vi "Do Core.vi"(8 "error in (no error)":errorcluster, 10 "Actor in":refnum<class "Actor.lvclass">, 11 "Ack Completion Long Exec Meth Msg in":refnum<class "Ack Completion with Error Msg.lvclass">) -> (0 "error out":errorcluster, 2 "Actor out":refnum<class "Actor.lvclass">)   [LabVIEW 2023, in "Async Methods Actor Example.lvlib" / "Ack Completion with Error Msg.lvclass"]
doc: "(<B>Filename</B>: Actor Framework.lvlib:Message.lvclass:Do.vi)\n\nDefines what a message does when it is received by an actor. Generally, a message instructs an actor to invoke one of its methods. By default, this method does nothing. A child class must override it to define behavior. Create a child class by using the Actor Framework Message Maker dialog box."
uses:
  Ack Completion with Error Msg.lvclass
  C:/Program Files/National Instruments/LabVIEW 2023/vi.lib/LS Instruments AG/Async Methods Actor/Async Methods Actor/Async Methods Actor Messages/Completion Notification Msg/Completion Notification Msg.lvclass
  <vilib>/ActorFramework/Actor/Actor.lvclass
  Async Methods Actor Example/Async Methods Actor Example.lvclass
  C:/Program Files/National Instruments/LabVIEW 2023/vi.lib/ActorFramework/Actor/Actor.lvclass
  <vilib>/LS Instruments AG/Async Methods Actor/Async Methods Actor/Async Methods Actor Messages/Completion Notification Msg/Completion Notification Data.ctl
  <vilib>/LS Instruments AG/Async Methods Actor/Async Methods Actor/Async Methods Actor Messages/Async Message/Async Message.lvclass
  <vilib>/LS Instruments AG/Async Methods Actor/Async Methods Actor/Async Methods Actor Messages/Completion Notification Msg/Completion Notification Msg.lvclass/Completion Notification Msg.ctl
  <vilib>/LS Instruments AG/Async Methods Actor/Async Methods Actor/Async Methods Actor Messages/Completion Notification Msg/Read Async Message.vi
  <vilib>/LS Instruments AG/Async Methods Actor/Async Methods Actor/Async Methods Actor Messages/Completion Notification Msg/Read Current Execution Count.vi
  <vilib>/LS Instruments AG/Async Methods Actor/Async Methods Actor/Async Methods Actor Messages/Completion Notification Msg/Completion Notification Msg.lvclass
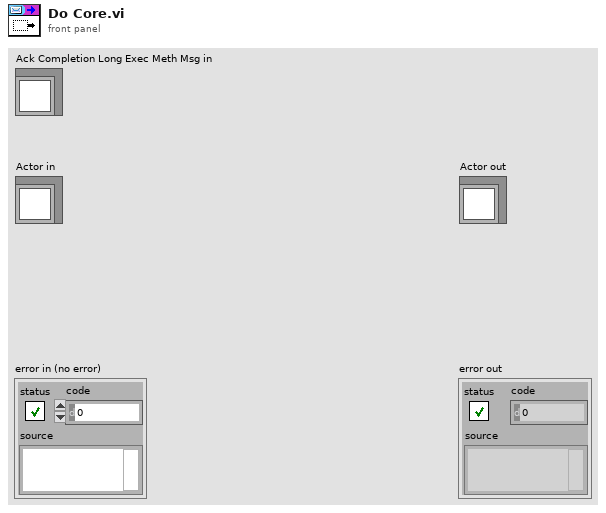
[diagram p1: front panel]
types:
  T1 = typedef "Async Methods Actor.lvlib/Completion Notification Msg.lvclass/Completion Notification Data.ctl" = cluster{"Async Message":refnum<class "Async Message.lvclass">, "Current Execution Count":u32}
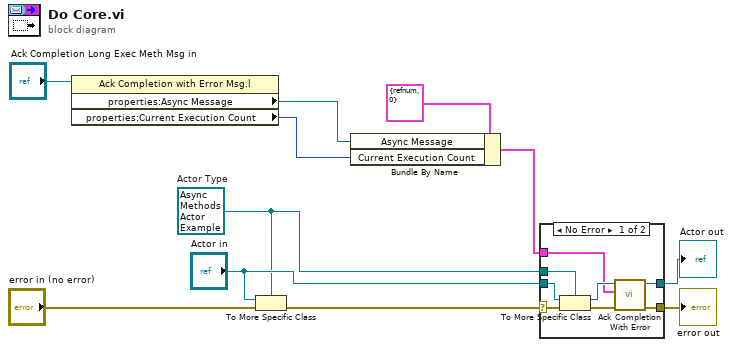
[diagram p0: block diagram]
diagram:
  w7 = refnum<class "Async Methods Actor Example.lvclass"> refnum  # Actor Type
  n1 = property class="Ack Completion with Error Msg.l"(reference="Ack Completion Long Exec Meth Msg in") -> ("properties:Async Message"=w3:refnum<class "Async Message.lvclass">, "properties:Current Execution Count"=w2:u32)  [unwired: 1 in, 2 out]
  n2 = To More Specific Class(target class=w7, reference="Actor in", error in="error in (no error)") -> (error out=w11:errorcluster)  [unwired: 1 out]
  n3 = Bundle By Name(cluster=T1 {"Async Message"=refnum, "Current Execution Count"=0} ("Completion Ack Data"), "Async Message"=w3, "Current Execution Count"=w2) -> (w4:T1)
  n4 = case shown="No Error" w11 {
    selector: w11 -> [w19 w21]
    tunnel: [w14 w21] -> w10
    tunnel: [w13 w20] -> w9
    tunnel: "Actor in" -> [w18 w20]
    tunnel: w7 -> [w17 _]
    tunnel: w4 -> [w12 _]
    frame No Error {
      n5 = To More Specific Class ("Actor Cast")(target class=w17, reference=w18, error in=w19) -> (specific class reference=w16:refnum<class "Async Methods Actor Example.lvclass">, error out=w15:errorcluster)
      n6 = call "Ack Completion With Error.vi"("error in (no error)"=w15, "Completion Ack Data"=w12, "Async Methods Actor Example in"=w16) -> ("error out"=w14:errorcluster, "Async Methods Actor Example out"=w13:refnum<class "Async Methods Actor Example.lvclass">)  [unwired: 7 in]
    }
    frame Error {
    }
  }
  "error out" <- w10
  "Actor out" <- w9
